vi "SysInfo-Restore Panel Position.vi"(0 "VI Refnum":refnum<vi>, 5 "Width":u32, 7 "Height":u32, 11 "error in (no error)":errorcluster) -> (4 "VI Refnum thru":refnum<vi>, 8 "Front Panel.WinBounds":T1, 15 "error out":errorcluster)   [LabVIEW 2020]
uses:
  <vilib>/Utility/miscctls.llb/LVRectTypeDef.ctl
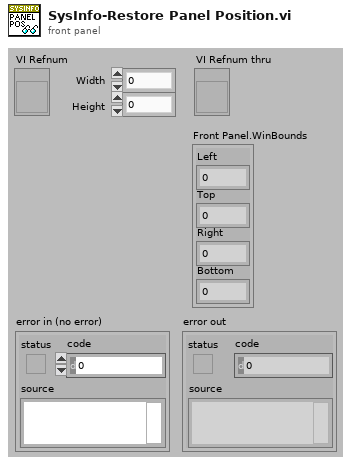
[diagram p1: front panel]
types:
  T1 = typedef "LVRectTypeDef.ctl" = cluster{"Left":i16, "Top":i16, "Right":i16, "Bottom":i16}
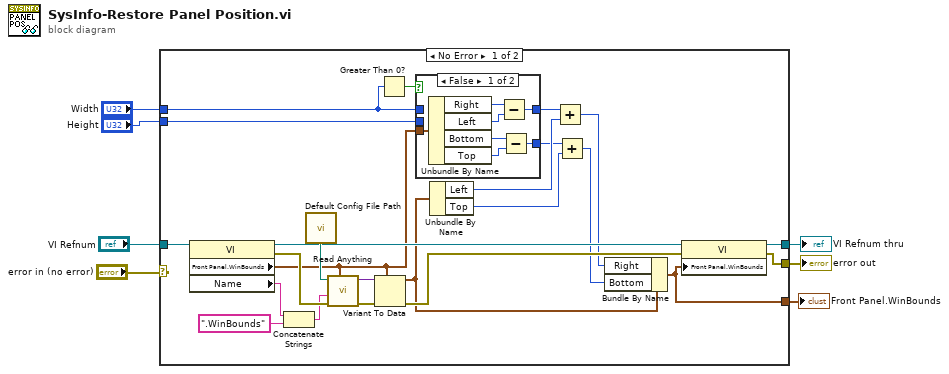
[diagram p0: block diagram]
diagram:
  n1 = case shown="No Error" "error in (no error)" {
    selector: "error in (no error)" -> [_ w42]
    tunnel: [w24 w42] -> w6
    tunnel: "VI Refnum" -> [w31 w41]
    tunnel: "Width" -> [w10 _]
    tunnel: "Height" -> [w12 _]
    tunnel: [w9 w41] -> w2
    tunnel: [w8 _] -> w1
    frame No Error {
      n2 = property class="VI"(reference=w31) -> (reference out=w25:refnum<vi>, error out=w29:errorcluster, "Front Panel.WinBounds"=w20:T1, "Name"=w23:string)  [unwired: 1 in]
      n3 = Concatenate Strings(w23, ".WinBounds" ("string")) -> (w22:string)
      n4 = call "Default Config File Path.vi"() -> ("Default config file name"=w30:path)
      n5 = call "Read Anything.vi"("Type of Anything"=w20, "Error In"=w29, "Section Name (Name of \"Type of Anything\")"=w22, "Path (dialog)"=w30) -> ("Error Out"=w28:errorcluster, "Anything"=w27:variant)  [unwired: 5 in, 1 out]
      n6 = Variant To Data(error in=w28, type=w20, Variant=w27) -> (data=w15:T1, error out=w26:errorcluster)
      n7 = Greater Than 0?(x=w10) -> (x > 0?=w11:bool)
      n8 = case shown="False" w11 {
        tunnel: w20 -> [w38 _]
        tunnel: [w33 w40] -> w19
        tunnel: [w32 w39] -> w17
        tunnel: w10 -> [_ w40]
        tunnel: w12 -> [_ w39]
        frame False {
          n9 = Unbundle By Name(w38) -> ("Right"=w37:i16, "Left"=w36:i16, "Bottom"=w35:i16, "Top"=w34:i16)
          n10 = Subtract(x=w37, y=w36) -> (x-y=w33:i16)
          n11 = Subtract(x=w35, y=w34) -> (x-y=w32:i16)
        }
        frame True {
        }
      }
      n12 = Unbundle By Name(w15) -> ("Left"=w18:i16, "Top"=w16:i16)
      n13 = Add(x=w19, y=w18) -> (x+y=w14:u32)
      n14 = Add(x=w17, y=w16) -> (x+y=w13:u32)
      n15 = Bundle By Name(cluster=w15, "Right"=w14, "Bottom"=w13) -> (w8:T1)
      n16 = property class="VI"(reference=w25, error in=w26, "Front Panel.WinBounds"=w8) -> (reference out=w9:refnum<vi>, error out=w24:errorcluster)
    }
    frame Error {
    }
  }
  "error out" <- w6
  "VI Refnum thru" <- w2
  "Front Panel.WinBounds" <- w1
